vi "波形转数组.vi"(11 "响应信号":waveform(dbl)) -> (3 "数组":string[][](array[string]))   [LabVIEW 2018]
uses:
  <vilib>/Waveform/WDTOps.llb/WDT Get Waveform Time Array DBL.vi
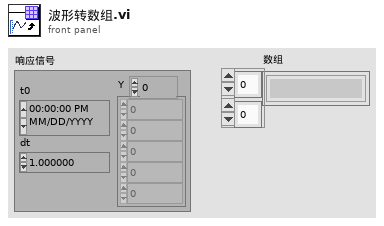
[diagram p1: front panel]
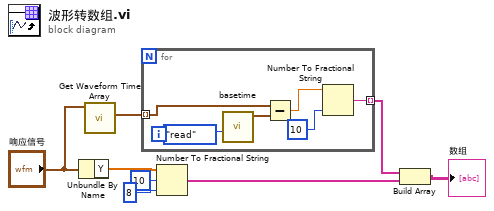
[diagram p0: block diagram]
diagram:
  n1 = Unbundle By Name("响应信号") -> ("Y"=w6:dbl[])
  n2 = call-poly <vilib>:"Get Waveform Time Array.vi"("waveform in"="响应信号") -> ("X array"=w5:timestamp[])  [unwired: 9 in, 1 out]
  n3 = for {
    tunnel: w5 -> [w12] mode=indexing
    tunnel: [w9] -> w1 mode=indexing
    n4 = call "basetime.vi"("枚举"=enum16{"write", "read"}."read") -> ("basetime"=w13:timestamp)  [unwired: 10 in]
    n5 = Subtract(x=w12, y=w13) -> (x-y=w11:dbl)
    n6 = Number To Fractional String(number=w11, precision (6)=i16 10 ("宽度(-)")) -> (F-format string=w9:string)  [unwired: 2 in]
  }
  n7 = Number To Fractional String(number=w6, width (-)=i16 10 ("宽度(-)"), precision (6)=i16 8 ("宽度(-)")) -> (F-format string=w3:string[])  [unwired: 1 in]
  n8 = Build Array(w1, w3) -> (→"数组":string[][])
